vi "Set Team names.vi"(8 "error in (no error)":errorcluster, 10 "Names":string[](array[string]), 11 "State Data in":T1) -> (0 "error out":errorcluster, 3 "State Data out":T1)   [LabVIEW 2025]
uses:
  State Data.ctl
  Team.ctl
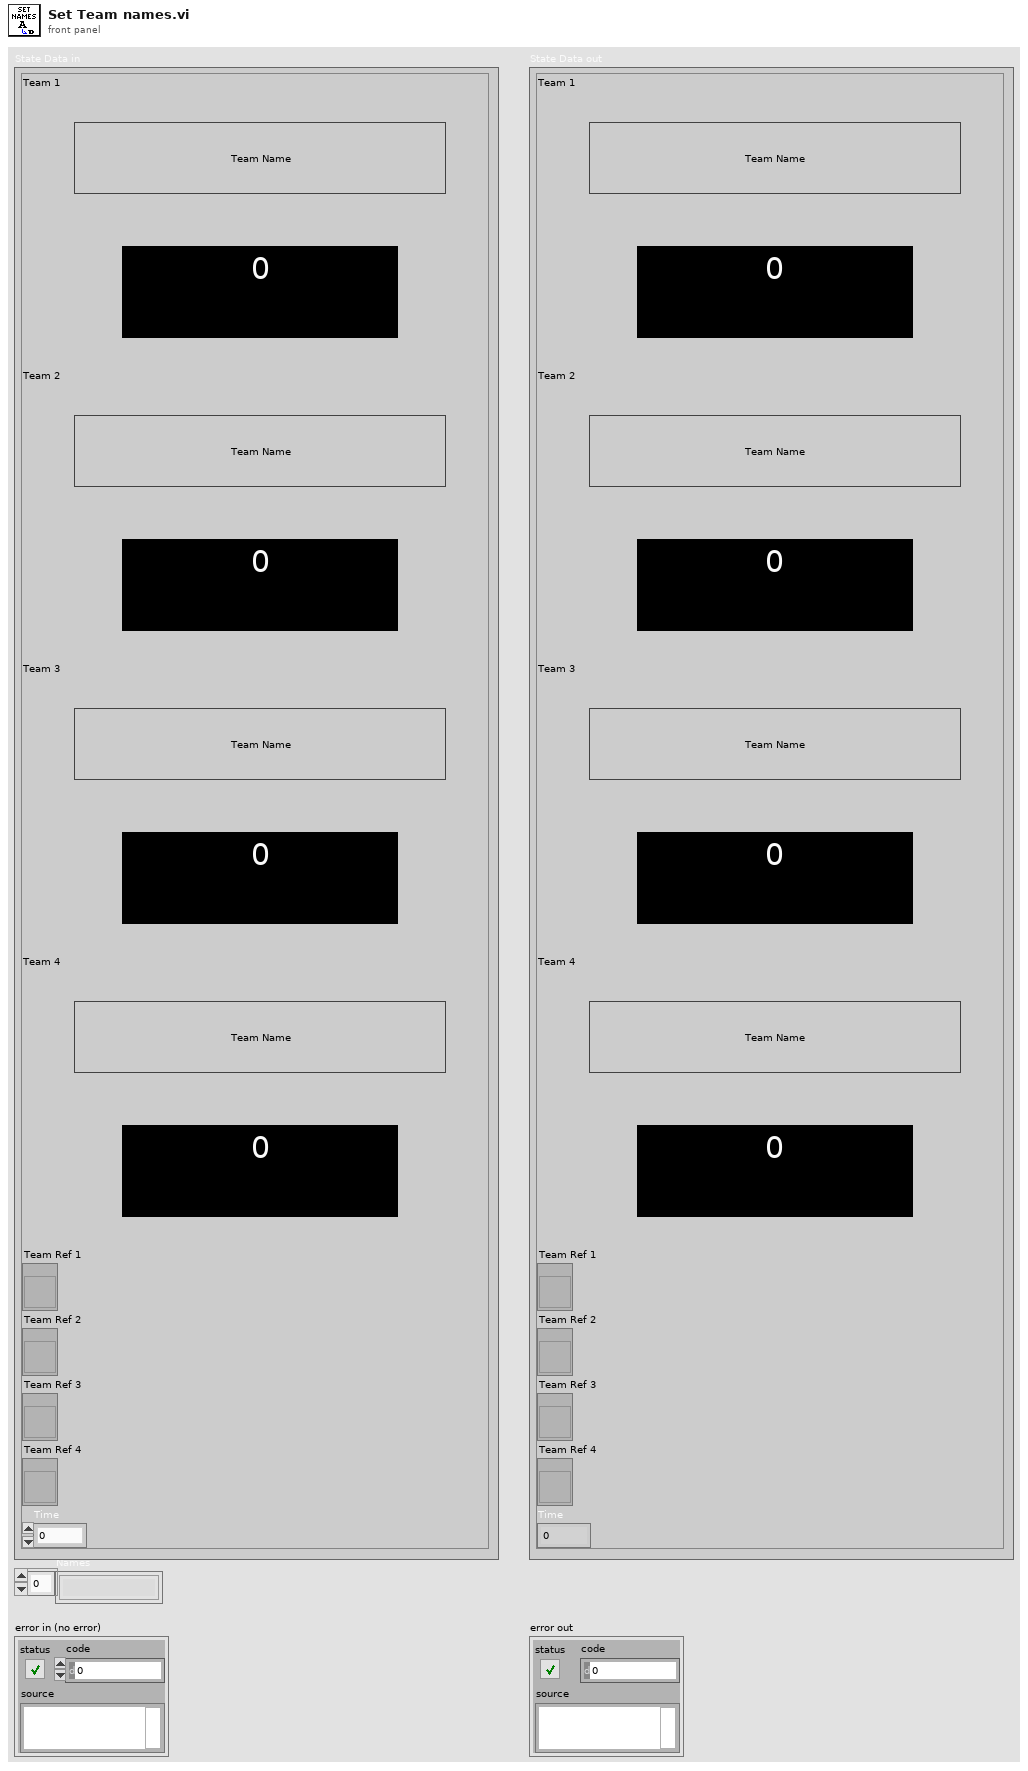
[diagram p1: front panel]
types:
  T1 = typedef "State Data.ctl" = cluster{"Team 1":T2, "Team 2":T2, "Team 3":T2, "Team 4":T2, "Team Ref 1":refnum<vi>, "Team Ref 2":refnum<vi>, "Team Ref 3":refnum<vi>, "Team Ref 4":refnum<vi>, "Time":i32}
  T2 = typedef "Team.ctl" = cluster{"ON":bool, "Name":bool, "Score":i32, "Split":string}
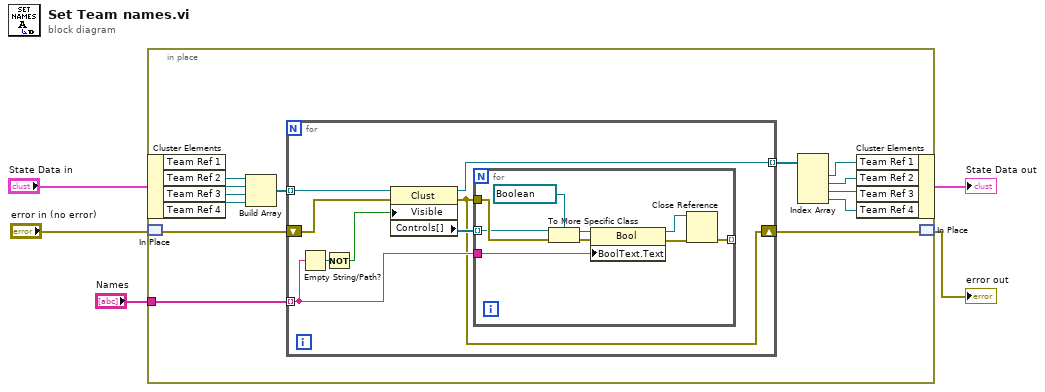
[diagram p0: block diagram]
diagram:
  n1 = in-place {
    in-place-border: "Names" -> [w12]
    n2 = in-place-cluster #1("State Data in") -> ("Team Ref 1"=w18:refnum<vi>, "Team Ref 2"=w17:refnum<vi>, "Team Ref 3"=w16:refnum<vi>, "Team Ref 4"=w15:refnum<vi>)
    n3 = in-place-match #2("error in (no error)") -> (w13:errorcluster)
    n4 = Build Array(w18, w17, w16, w15) -> (w14:refnum<vi>[])
    n5 = for {
      tunnel: w14 -> [w26] mode=indexing
      tunnel: w12 -> [w21] mode=indexing
      shift-right: [w20] -> w11
      shift-left: w13 -> [w25]
      tunnel: [w19] -> w10 mode=indexing
      n6 = Empty String/Path?(string/path=w21) -> (empty?=w24:bool)
      n7 = Not(x=w24) -> (.not. x?=w23:bool)
      n8 = property class="Clust"(reference=w26, error in=w25, "Visible"=w23) -> (reference out=w19:refnum<vi>, error out=w20:errorcluster, "Controls[]"=w22:refnum<vi>[])
      n9 = for {
        tunnel: w22 -> [w27] mode=indexing
        tunnel: w20 -> [w34]
        tunnel: w21 -> [w31]
        tunnel: [w28] -> _ mode=indexing
        n10 = To More Specific Class(target class=refnum<vi> refnum ("Name"), reference=w27, error in=w34) -> (specific class reference=w33:refnum<vi>, error out=w32:errorcluster)
        n11 = property class="Bool"(reference=w33, error in=w32, "BoolText.Text"=w31) -> (reference out=w29:refnum<vi>, error out=w30:errorcluster)
        n12 = Close Reference(reference=w29, error in (no error)=w30) -> (error out=w28:errorcluster)
      }
    }
    n13 = Index Array(array=w10) -> (element #1=w9:refnum<vi>, element #2=w8:refnum<vi>, element #3=w7:refnum<vi>, element #4=w6:refnum<vi>)  [unwired: 4 in]
    n14 = in-place-cluster #1("Team Ref 1"=w9, "Team Ref 2"=w8, "Team Ref 3"=w7, "Team Ref 4"=w6) -> (→"State Data out":T1)
    n15 = in-place-match #2(w11) -> (→"error out":errorcluster)
  }
